vi "Default UDP.vi"() -> (3 "String":string)   [LabVIEW 2016]
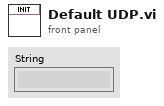
[diagram p1: front panel]
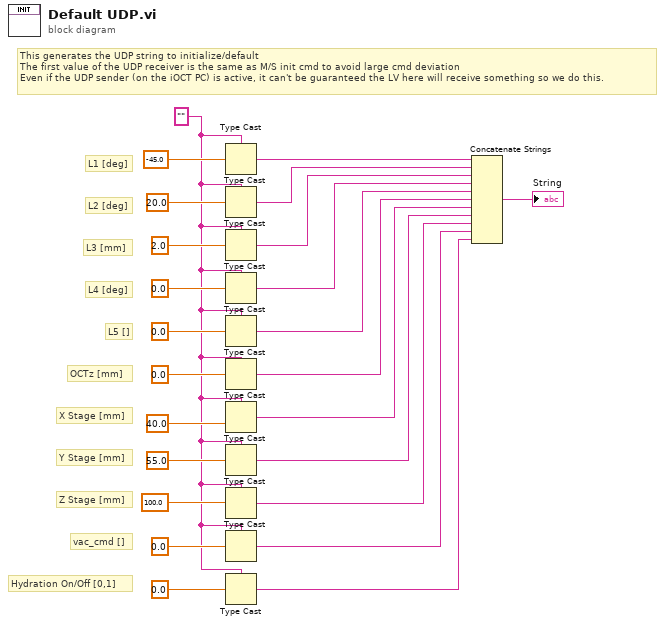
[diagram p0: block diagram]
diagram:
  w4 = "" ("data in")
  # "This generates the UDP string to initialize/default \nThe first value of the UDP receiver is the same as M/S init cmd to avoid large cmd deviation\nEven if the UDP sender (on the iOCT PC) is active, it can't be guaranteed the LV here will receive something so we do this."
  # "Hydration On/Off [0,1]"
  # "vac_cmd []"
  # "Z Stage [mm]"
  # "Y Stage [mm]"
  # "X Stage [mm]"
  # "OCTz [mm]"
  # "L5 []"
  # "L4 [deg]"
  # "L3 [mm]"
  # "L2 [deg]"
  # "L1 [deg]"
  n1 = Type Cast(type=w4, x=sgl -45.0 ("number")) -> (*(type *) &x=w1:string)
  n2 = Type Cast(type=w4, x=sgl 20.0 ("number")) -> (*(type *) &x=w3:string)
  n3 = Type Cast(type=w4, x=sgl 2.0 ("number")) -> (*(type *) &x=w2:string)
  n4 = Type Cast(type=w4, x=sgl 0.0 ("number")) -> (*(type *) &x=w5:string)
  n5 = Type Cast(type=w4, x=sgl 0.0 ("number")) -> (*(type *) &x=w6:string)
  n6 = Type Cast(type=w4, x=sgl 0.0 ("number")) -> (*(type *) &x=w7:string)
  n7 = Type Cast(type=w4, x=sgl 40.0 ("number")) -> (*(type *) &x=w8:string)
  n8 = Type Cast(type=w4, x=sgl 55.0 ("number")) -> (*(type *) &x=w9:string)
  n9 = Type Cast(type=w4, x=sgl 100.0 ("number")) -> (*(type *) &x=w10:string)
  n10 = Type Cast(type=w4, x=sgl 0.0 ("number")) -> (*(type *) &x=w11:string)
  n11 = Type Cast(type=w4, x=sgl 0.0 ("number")) -> (*(type *) &x=w12:string)
  n12 = Concatenate Strings(w1, w3, w2, w5, w6, w7, w8, w9, w10, w11, w12) -> (→"String":string)
